vi "LaserScan2ROSMsg.vi"(10 "LaserScan":T1, 11 "msg in":string) -> (3 "msg out":string)   [LabVIEW 2014]
uses:
  LaserScan.ctl
  <userlib>/ROS for LabVIEW Software/ROS/MessageBuilding/std_msgs/subs/u8Scalar.vi
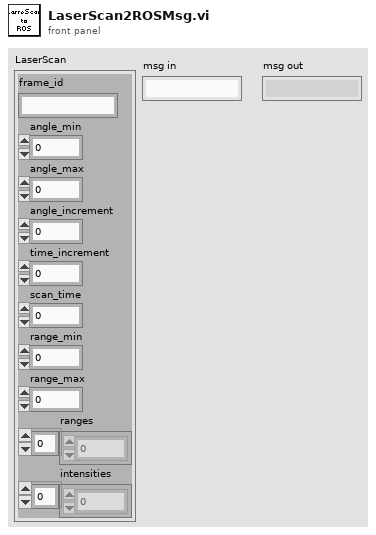
[diagram p1: front panel]
types:
  T1 = typedef "LaserScan.ctl" = cluster{"frame_id":string, "angle_min":dbl, "angle_max":dbl, "angle_increment":dbl, "time_increment":dbl, "scan_time":dbl, "range_min":dbl, "range_max":dbl, "ranges":dbl[], "intensities":dbl[]}
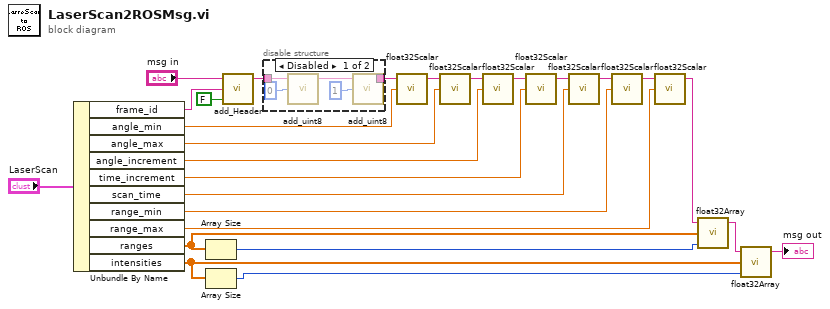
[diagram p0: block diagram]
diagram:
  n1 = Unbundle By Name("LaserScan") -> ("frame_id"=w25:string, "angle_min"=w23:dbl, "angle_max"=w22:dbl, "angle_increment"=w21:dbl, "time_increment"=w20:dbl, "scan_time"=w19:dbl, "range_min"=w18:dbl, "range_max"=w17:dbl, "ranges"=w15:dbl[], "intensities"=w9:dbl[])
  n2 = Array Size(array=w15) -> (size(s)=w14:i32)
  n3 = Array Size(array=w9) -> (size(s)=w1:i32)
  n4 = call <userlib>:"add_Header.vi"("reset seq?"=FALSE, "frame_id"=w25, "msg in"="msg in") -> ("msg out"=w12:string)  [unwired: 2 in]
  n5 = disable-structure shown="Disabled" {
    disable-tunnel: w12 -> [w28 w32]
    disable-tunnel: [w27 w32] -> w10
    frame Disabled {
      n6 = call-poly <userlib>:"add_uint8.vi"("Numeric"=u8 0, "msg in"=w28) -> ("msg out"=w31:string)  [unwired: 3 in]
      n7 = call-poly <userlib>:"add_uint8.vi"("Numeric"=u8 1, "msg in"=w31) -> ("msg out"=w27:string)  [unwired: 3 in]
    }
    frame Enabled {
    }
  }
  n8 = call <userlib>:"float32Scalar.vi"("Numeric"=w23, "msg in"=w10) -> ("msg out"=w8:string)  [unwired: 3 in]
  n9 = call <userlib>:"float32Scalar.vi"("Numeric"=w22, "msg in"=w8) -> ("msg out"=w7:string)  [unwired: 3 in]
  n10 = call <userlib>:"float32Scalar.vi"("Numeric"=w21, "msg in"=w7) -> ("msg out"=w6:string)  [unwired: 3 in]
  n11 = call <userlib>:"float32Scalar.vi"("Numeric"=w20, "msg in"=w6) -> ("msg out"=w5:string)  [unwired: 3 in]
  n12 = call <userlib>:"float32Scalar.vi"("Numeric"=w19, "msg in"=w5) -> ("msg out"=w4:string)  [unwired: 3 in]
  n13 = call <userlib>:"float32Scalar.vi"("Numeric"=w18, "msg in"=w4) -> ("msg out"=w3:string)  [unwired: 3 in]
  n14 = call <userlib>:"float32Scalar.vi"("Numeric"=w17, "msg in"=w3) -> ("msg out"=w16:string)  [unwired: 3 in]
  n15 = call <userlib>:"float32Array.vi"("Array Length"=w14, "Array"=w15, "msg in"=w16) -> ("msg out"=w2:string)  [unwired: 2 in]
  n16 = call <userlib>:"float32Array.vi"("Array Length"=w1, "Array"=w9, "msg in"=w2) -> ("msg out"=→"msg out":string)  [unwired: 2 in]
